vi "snl_test.vi"() -> ()   [LabVIEW 2019]
uses:
  <vilib>/Utility/file.llb/Read Delimited Spreadsheet (DBL).vi
panel:
  out "snlData":dbl[][](array[numeric])
  out "trans force":dbl[](array[numeric])
  in  "max foce (mN)":dbl
  in  "min force (mN)":dbl
  out "calc PW":dbl
  in  "force ref":dbl
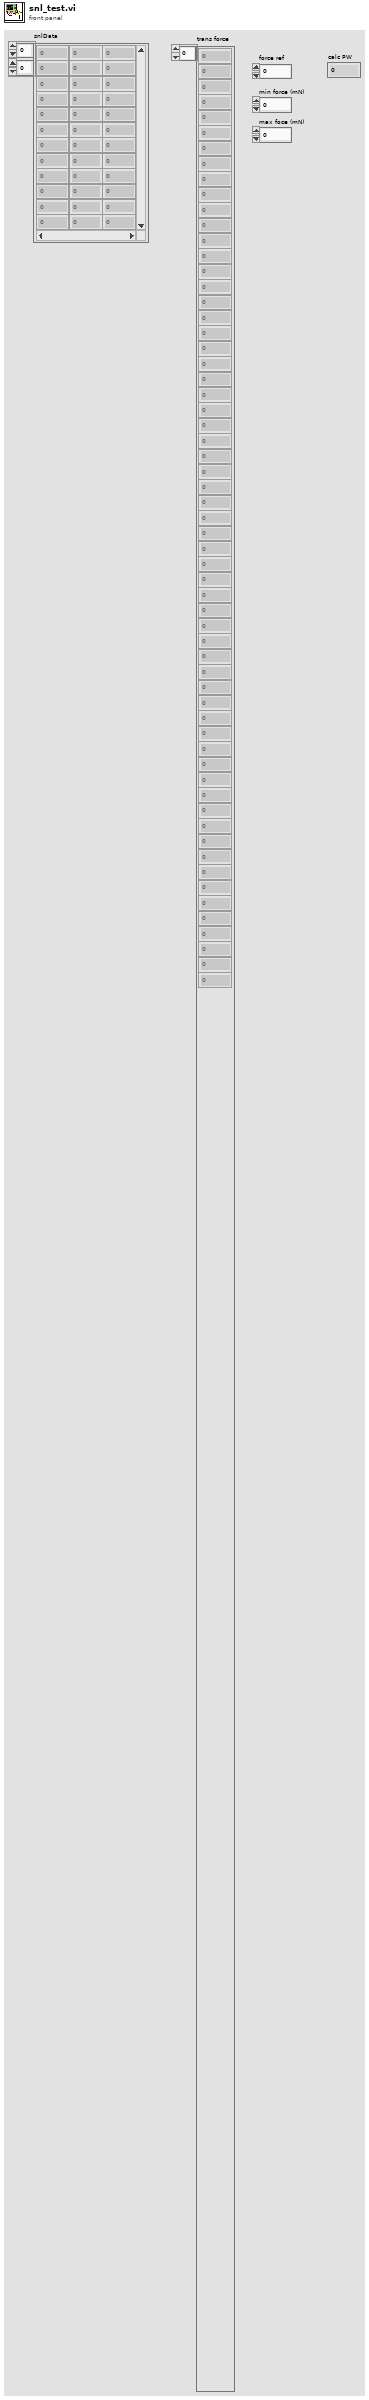
[diagram p1: front panel]
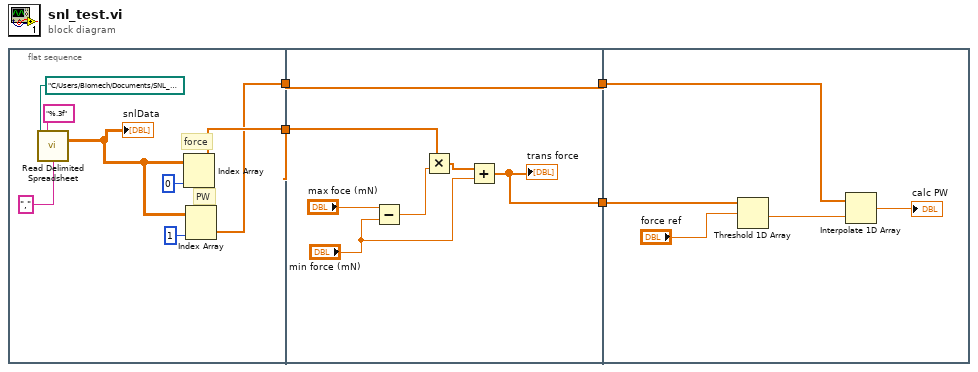
[diagram p0: block diagram]
diagram:
  n1 = flat-sequence {
    tunnel: [w6] -> w3
    tunnel: [w5] -> w2
    tunnel: [w15] -> w4
    tunnel: w3 -> [w14]
    tunnel: w2 -> [w13]
    tunnel: [w13] -> w1
    tunnel: w4 -> [w21]
    tunnel: w1 -> [w20]
    frame #0 {
      # "PW"
      # "force"
      n2 = call-poly <vilib>:"Read Delimited Spreadsheet.vi"("file path (dialog if empty)"=path "C:/Users/Biomech/Documents/SNL_matlab.txt", "format (%.3f)"="%.3f", "delimiter (\\t)"="," ("delimiter (\\t)")) -> ("all rows"=w8:dbl[][])  [unwired: 7 in, 5 out]
      "snlData" <- w8
      n3 = Index Array(array=w8, index (col)=0 ("disabled index (col)")) -> (element=w6:dbl[])  [unwired: 1 in]
      n4 = Index Array(array=w8, index (col)=1 ("disabled index (col)")) -> (element=w5:dbl[])  [unwired: 1 in]
    }
    frame #1 {
      n5 = Subtract(x="max foce (mN)", y="min force (mN)") -> (x-y=w18:dbl)
      n6 = Multiply(x=w14, y=w18) -> (x*y=w17:dbl[])
      n7 = Add(x=w17, y="min force (mN)") -> (x+y=w15:dbl[])
      "trans force" <- w15
    }
    frame #2 {
      n8 = Threshold 1D Array(2:"force ref", 3:w21) -> (0:w23:dbl)  [unwired: 1 in]
      n9 = Interpolate 1D Array(1:w23, 2:w20) -> (0:→"calc PW":dbl)
    }
  }
